vi "run_tests_of_given_path.vi"(11 "Command Line":string[](array[string])) -> (2 "stdout | stderr":string, 3 "Return Code":i32)   [LabVIEW 2020]
uses:
  <vilib>/Utility/error.llb/DialogType.ctl
  <vilib>/Utility/error.llb/Error Cluster From Error Code.vi
  <vilib>/ErrorRing/Error Ring.xnode
panel:
  out "error out":errorcluster
  in  "error in (no error)":errorcluster
  in  "Tests":path[](array[path])=[path "C:/ar/_work/measurementlink-labview/measurementlink-labview/Source/Tests/Tests.Runtime/Measurement Server/Discovery/test_DiscoveryServiceNotRunning_LaunchDiscoveryService_DiscoveryServiceStarted.vi", path "C:/ar/_work/measurementlink-labview/measurementlink-labview/Source/Tests/Tests.Runtime/Measurement Server/Session Management/Session Reservation/test_SessionManagerWrapper_StopSessionManagementService_WrapperMethodsWorkWithoutError.vi", path "C:/ar/_work/measurementlink-labview/measurementlink-labview/Source/Tests/Tests.Runtime/Measurement Server/Discovery/test_DiscoveryWrapper_StopDiscoveryService_WrapperMethodsWorkWithoutError.vi", path "C:/ar/_work/measurementlink-labview/measurementlink-labview/Source/Tests/Tests.Runtime/Measurement Server/Initialize Sessions/test_DCPowerInstrument_InitializeSessionsWithUnregisteredSessionsReserved_RemoteSessionsInitialized.vi"]
  out "Full Report":string
  out "All Tests Passed":bool
  out "Detailed Test Results path":path
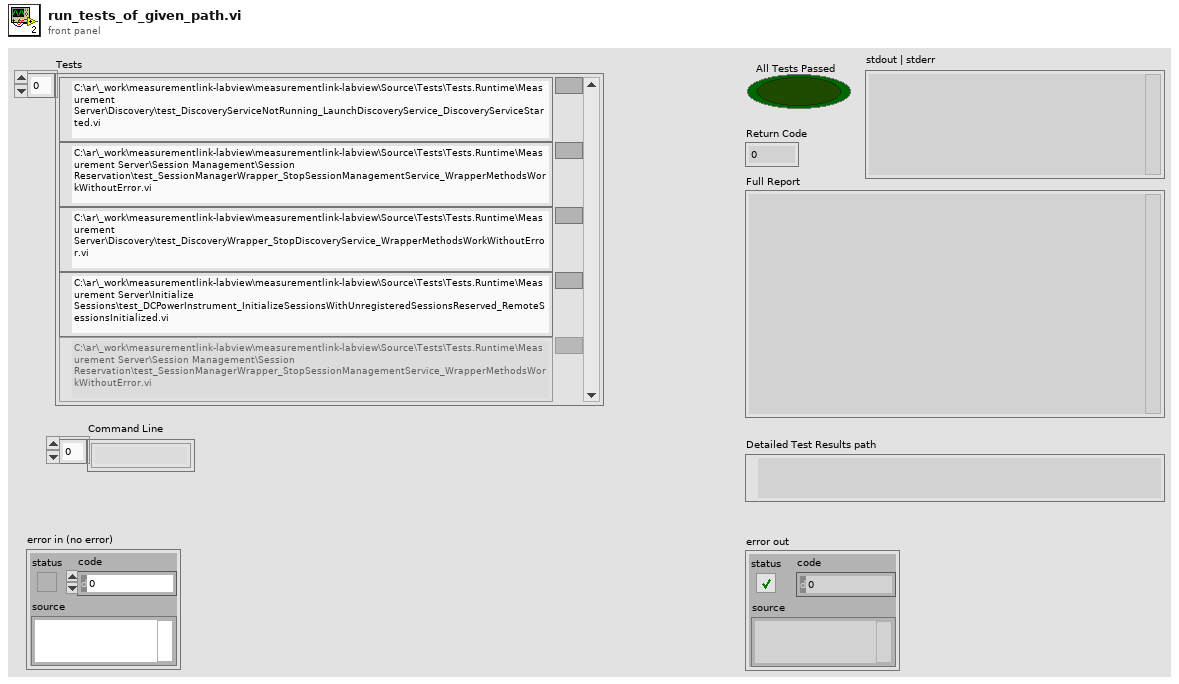
[diagram p1: front panel]
types:
  T1 = enum16{"open", "replace", "create", "open or create", "replace or create", "replace or create with confirmation"}
  T2 = typedef "DialogType.ctl" = u16
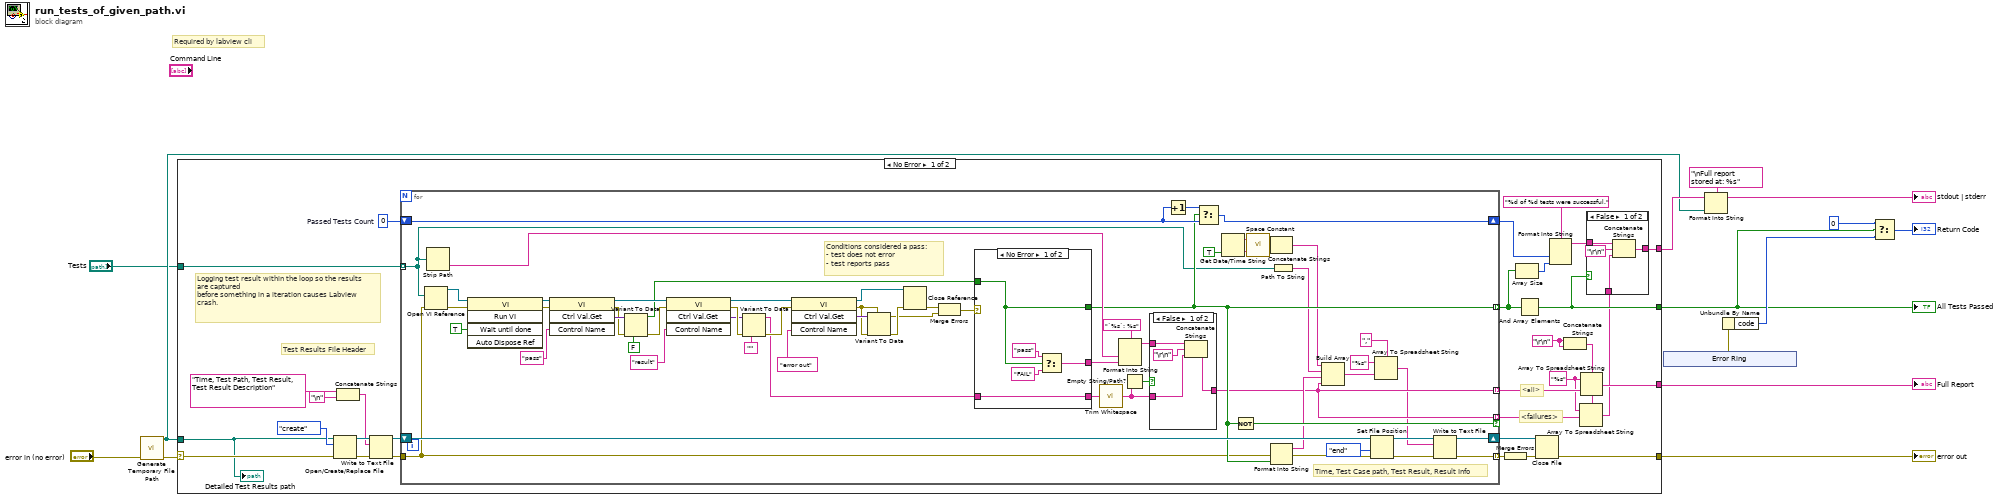
[diagram p0: block diagram]
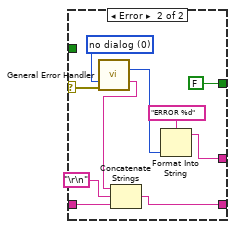
[diagram p4: hidden frame]
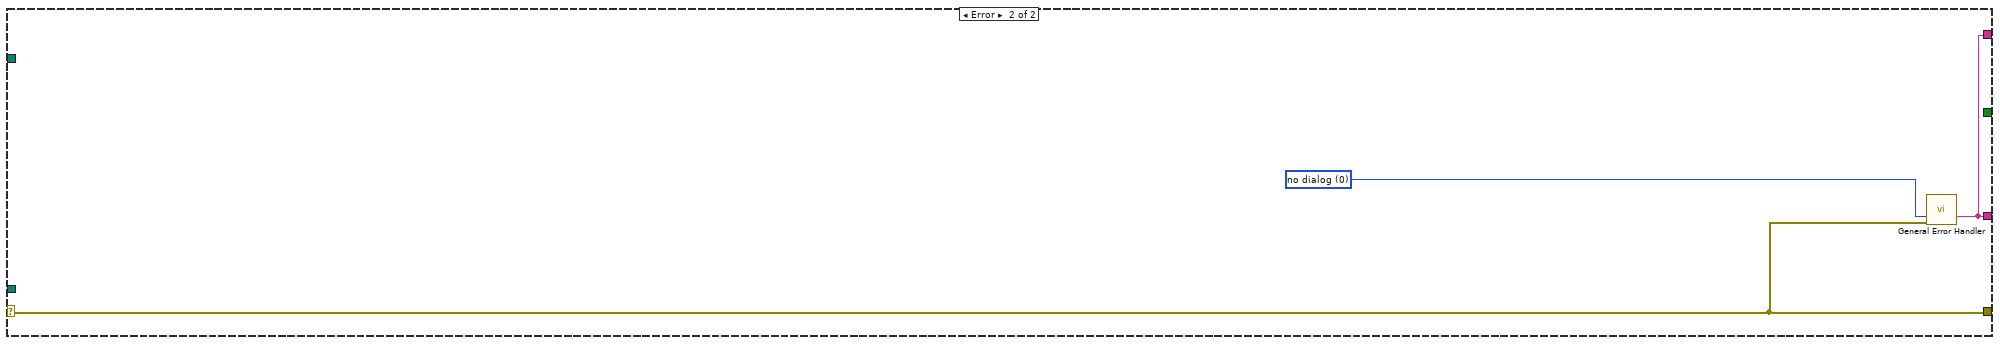
[diagram p5: hidden frame]
diagram:
  # "Required by labview cli"
  n1 = call <vilib>:"Generate Temporary File Path.vi"("error in (no error)"="error in (no error)") -> ("error out"=w9:errorcluster, "Unique Temporary File Path"=w8:path)  [unwired: 9 in]
  n2 = case shown="No Error" w9 {
    selector: w9 -> [w16 w132]
    tunnel: "Tests" -> [w44 _]
    tunnel: [w17 w132] -> w5
    tunnel: [w37 _] -> w3
    tunnel: [w34 w130] -> w13
    tunnel: [w35 w130] -> w11
    tunnel: w8 -> [w15 _]
    frame No Error {
      w41 = 0  # Passed Tests Count
      w30 = "%s" ("format string")
      w43 = "\r\n"
      # "Logging test result within the loop so the results are captured\nbefore something in a iteration causes Labview crash."
      # "Test Results File Header"
      # "<failures>"
      # "<all>"
      n3 = Open/Create/Replace File(file path (use dialog)=w15, error in=w16, operation (0:open)=T1."create") -> (refnum out=w24:refnum<file>, error out=w23:errorcluster)  [unwired: 3 in, 1 out]
      n4 = Concatenate Strings("Time, Test Path, Test Result, Test Result Description" ("text"), "\n") -> (w19:string)
      n5 = Write to Text File(file (use dialog)=w24, text=w19, error in=w23) -> (refnum out=w21:refnum<file>, error out=w22:errorcluster)  [unwired: 1 in, 1 out]
      n6 = for {
        tunnel: w44 -> [w53] mode=indexing
        tunnel: w22 -> [w50]
        tunnel: [w61] -> w39 mode=indexing
        tunnel: [w59] -> w33 mode=indexing
        tunnel: [w59] -> w32 mode=indexing if=w76
        shift-right: [w63] -> w40
        shift-left: w41 -> [w74]
        tunnel: [w70] -> w27 mode=indexing
        shift-right: [w69] -> w28
        shift-left: w21 -> [w62]
        # "Time, Test Case path, Test Result, Result Info"
        # "Conditions considered a pass:\n- test does not error\n- test reports pass"
        n7 = Open VI Reference(vi path=w53, error in (no error)=w50) -> (vi reference=w109:refnum<vi>, error out=w108:errorcluster)  [unwired: 4 in]
        n8 = Strip Path(path=w53) -> (name=w73:string)  [unwired: 1 out]
        n9 = invoke class="VI" method="Run VI"(reference=w109, error in=w108, "Wait until done"=TRUE ("Wait Until Done")) -> (reference out=w106:refnum<vi>, error out=w105:errorcluster)  [unwired: 2 in, 3 out]
        n10 = invoke class="VI" method="Ctrl Val.Get"(reference=w106, error in=w105, "Control Name"="pass") -> (reference out=w95:refnum<vi>, error out=w102:errorcluster, "Get Control Value Variant"=w103:variant)  [unwired: 1 in, 1 out]
        n11 = Variant To Data(error in=w102, type=FALSE, Variant=w103) -> (data=w84:bool, error out=w99:errorcluster)
        n12 = invoke class="VI" method="Ctrl Val.Get"(reference=w95, error in=w99, "Control Name"="result") -> (reference out=w90:refnum<vi>, error out=w100:errorcluster, "Get Control Value Variant"=w97:variant)  [unwired: 1 in, 1 out]
        n13 = Variant To Data(error in=w100, type="", Variant=w97) -> (data=w81:string, error out=w93:errorcluster)
        n14 = invoke class="VI" method="Ctrl Val.Get"(reference=w90, error in=w93, "Control Name"="error out") -> (reference out=w89:refnum<vi>, error out=w91:errorcluster, "Get Control Value Variant"=w94:variant)  [unwired: 1 in, 1 out]
        n15 = Variant To Data(error in=w91, type=w91, Variant=w94) -> (data=w86:errorcluster, error out=w92:errorcluster)
        n16 = Close Reference(reference=w89, error in (no error)=w92) -> (error out=w87:errorcluster)
        n17 = Merge Errors(w87, w86) -> (w85:errorcluster)
        n18 = case shown="No Error" w85 {
          selector: w85 -> [_ w127]
          tunnel: w84 -> [w117 _]
          tunnel: [w116 w124] -> w82
          tunnel: [w117 FALSE] -> w61
          tunnel: w81 -> [w115 w123]
          tunnel: [w115 w122] -> w80
          frame No Error {
            n19 = Select(t="pass" ("Control Name"), s=w117, f="FAIL" ("Control Name")) -> (s? t:f=w116:string)
          }
          frame Error {
            w128 = T2 0 items=["no dialog", "OK message", "continue or stop message", "OK message + warnings", "continue/stop + warnings"] ("type of dialog (OK msg:1)")
            n20 = call <vilib>:"General Error Handler.vi"("type of dialog (OK msg:1)"=w128, "error in (no error)"=w127) -> ("code out"=w126:i32, "message"=w121:string)  [unwired: 9 in, 3 out]
            n21 = Concatenate Strings(w121, "\r\n", w123) -> (w122:string)
            n22 = Format Into String(format string="ERROR %d", w126) -> (resulting string=w124:string)  [unwired: 2 in, 1 out]
          }
        }
        n23 = call <vilib>:"Trim Whitespace.vi"("string"=w80) -> ("trimmed string"=w79:string)  [unwired: 1 in]
        n24 = Format Into String(format string="`%s`: %s" ("Control Name"), w73, w82) -> (resulting string=w77:string)  [unwired: 2 in, 1 out]
        n25 = Empty String/Path?(string/path=w79) -> (empty?=w78:bool)
        n26 = case shown="False" w78 {
          tunnel: w79 -> [w112 _]
          tunnel: w77 -> [w113 w114]
          tunnel: [w111 w114] -> w59
          frame False {
            n27 = Concatenate Strings(w113, "\r\n", w112) -> (w111:string)
          }
          frame True {
          }
        }
        n28 = Increment(x=w74) -> (x+1=w75:i32)
        n29 = Select(t=w75, s=w61, f=w74) -> (s? t:f=w63:i32)
        n30 = Get Date/Time String(want seconds? (F)=TRUE) -> (date string=w66:string, time string=w64:string)  [unwired: 2 in]
        n31 = Not(x=w61) -> (.not. x?=w76:bool)
        n32 = call <vilib>:"Space Constant.vi"() -> ("String"=w65:string)
        n33 = Concatenate Strings(w66, w65, w64) -> (w54:string)
        n34 = Format Into String(error in=w50, w61) -> (resulting string=w60:string, error out=w51:errorcluster)  [unwired: 2 in]
        n35 = Path To String(path=w53) -> (string=w52:string)
        n36 = Build Array(w54, w52, w60, w59) -> (w58:string[])
        n37 = Set File Position(refnum=w62, from (0:start)=enum16{"start", "end", "current"}."end", error in=w51) -> (refnum out=w71:refnum<file>, error out=w72:errorcluster)  [unwired: 1 in]
        n38 = Array To Spreadsheet String(delimiter (Tab)="," ("format string"), array=w58, 3:"%s" ("format string")) -> (spreadsheet string=w55:string)
        n39 = Write to Text File(file (use dialog)=w71, text=w55, error in=w72) -> (refnum out=w69:refnum<file>, error out=w70:errorcluster)  [unwired: 1 in, 1 out]
      }
      n40 = Merge Errors(w27) -> (w26:errorcluster)
      n41 = Array Size(array=w39) -> (size(s)=w38:i32)
      n42 = And Array Elements(Boolean array=w39) -> (logical AND=w37:bool)
      n43 = Close File(refnum=w28, error in=w26) -> (error out=w17:errorcluster)  [unwired: 1 out]
      n44 = Format Into String(format string="%d of %d tests were successful." ("Control Name"), w40, w38) -> (resulting string=w36:string)  [unwired: 2 in, 1 out]
      n45 = Concatenate Strings(w43, w43) -> (w31:string)
      n46 = Array To Spreadsheet String(delimiter (Tab)=w31, array=w32, 3:w30) -> (spreadsheet string=w29:string)
      n47 = Array To Spreadsheet String(delimiter (Tab)=w31, array=w33, 3:w30) -> (spreadsheet string=w34:string)
      n48 = case shown="False" w37 {
        tunnel: w36 -> [w48 w49]
        tunnel: [w45 w49] -> w35
        tunnel: w29 -> [w46 _]
        frame False {
          n49 = Concatenate Strings(w48, "\r\n", w46) -> (w45:string)
        }
        frame True {
        }
      }
      "Detailed Test Results path" <- w15
    }
    frame Error {
      w131 = T2 0 items=["no dialog", "OK message", "continue or stop message", "OK message + warnings", "continue/stop + warnings"] ("type of dialog (OK msg:1)")
      n50 = call <vilib>:"General Error Handler.vi"("type of dialog (OK msg:1)"=w131, "error in (no error)"=w132) -> ("message"=w130:string)  [unwired: 9 in, 4 out]
    }
  }
  "All Tests Passed" <- w3
  "Full Report" <- w13
  "error out" <- w5
  n51 = xnode "Error Ring"() -> ("error out"=w12:errorcluster)
  n52 = Format Into String(format string="\nFull report stored at: %s" ("Control Name"), initial string=w11, w8) -> (resulting string=→"stdout | stderr":string)  [unwired: 1 in, 1 out]
  n53 = Unbundle By Name(w12) -> ("code"=w4:i32)
  n54 = Select(t=0, s=w3, f=w4) -> (s? t:f=→"Return Code":i32)
